vi "Periodic Tasks.vi"(8 "error in":errorcluster) -> ()   [LabVIEW 2017]
doc: "This VI runs in parallel to other robot code. It can contain as many user-defined periodic loops as you need. These can carry out PID or other sorts of timed response."
uses:
  <vilib>/Rock Robotics/WPI/Utilities/WPI_GetSetVariantRefNum.vi
  Robot Global Data.vi
  <vilib>/Rock Robotics/Network Tables/NT Write Number.vi
  <vilib>/Rock Robotics/Network Tables/NT Write Boolean.vi
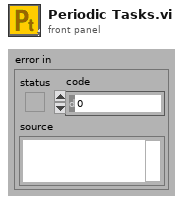
[diagram p1: front panel]
types:
  T1 = typedef "WPI_JoystickDevRef.ctl" = cluster{"Device":T2}
  T2 = typedef "WPI_JoystickDeviceEnum.ctl" = enum16{"USB 0", "USB 1", "USB 2", "USB 3", "USB 4", "USB 5"}
  T3 = typedef "WPI_GyroDevRef.ctl" = cluster{"DevStatus":errorcluster, "Analog Channel":T4, "Gain (VoltsPerDegree/Second)":dbl, "Gyro Type":enum16{"Analog", "XRS450"}, "Handle":i32, "SPI Bus":T5, "Device Found":bool, "Sample Rate":dbl, "Calibrate On Open":bool, "Offset":dbl}
  T4 = typedef "FPGA_AIChannel.ctl" = enum8{"AI 0", "AI 1", "AI 2", "AI 3", "AI MXP 0", "AI MXP 1", "AI MXP 2", "AI MXP 3", "Invalid"}
  T5 = typedef "spi_bus.ctl" = enum16{"SPI On-Board, CS0", "SPI On-Board, CS1", "SPI On-Board, CS2", "SPI On-Board, CS3", "SPI MXP", "Invalid"}
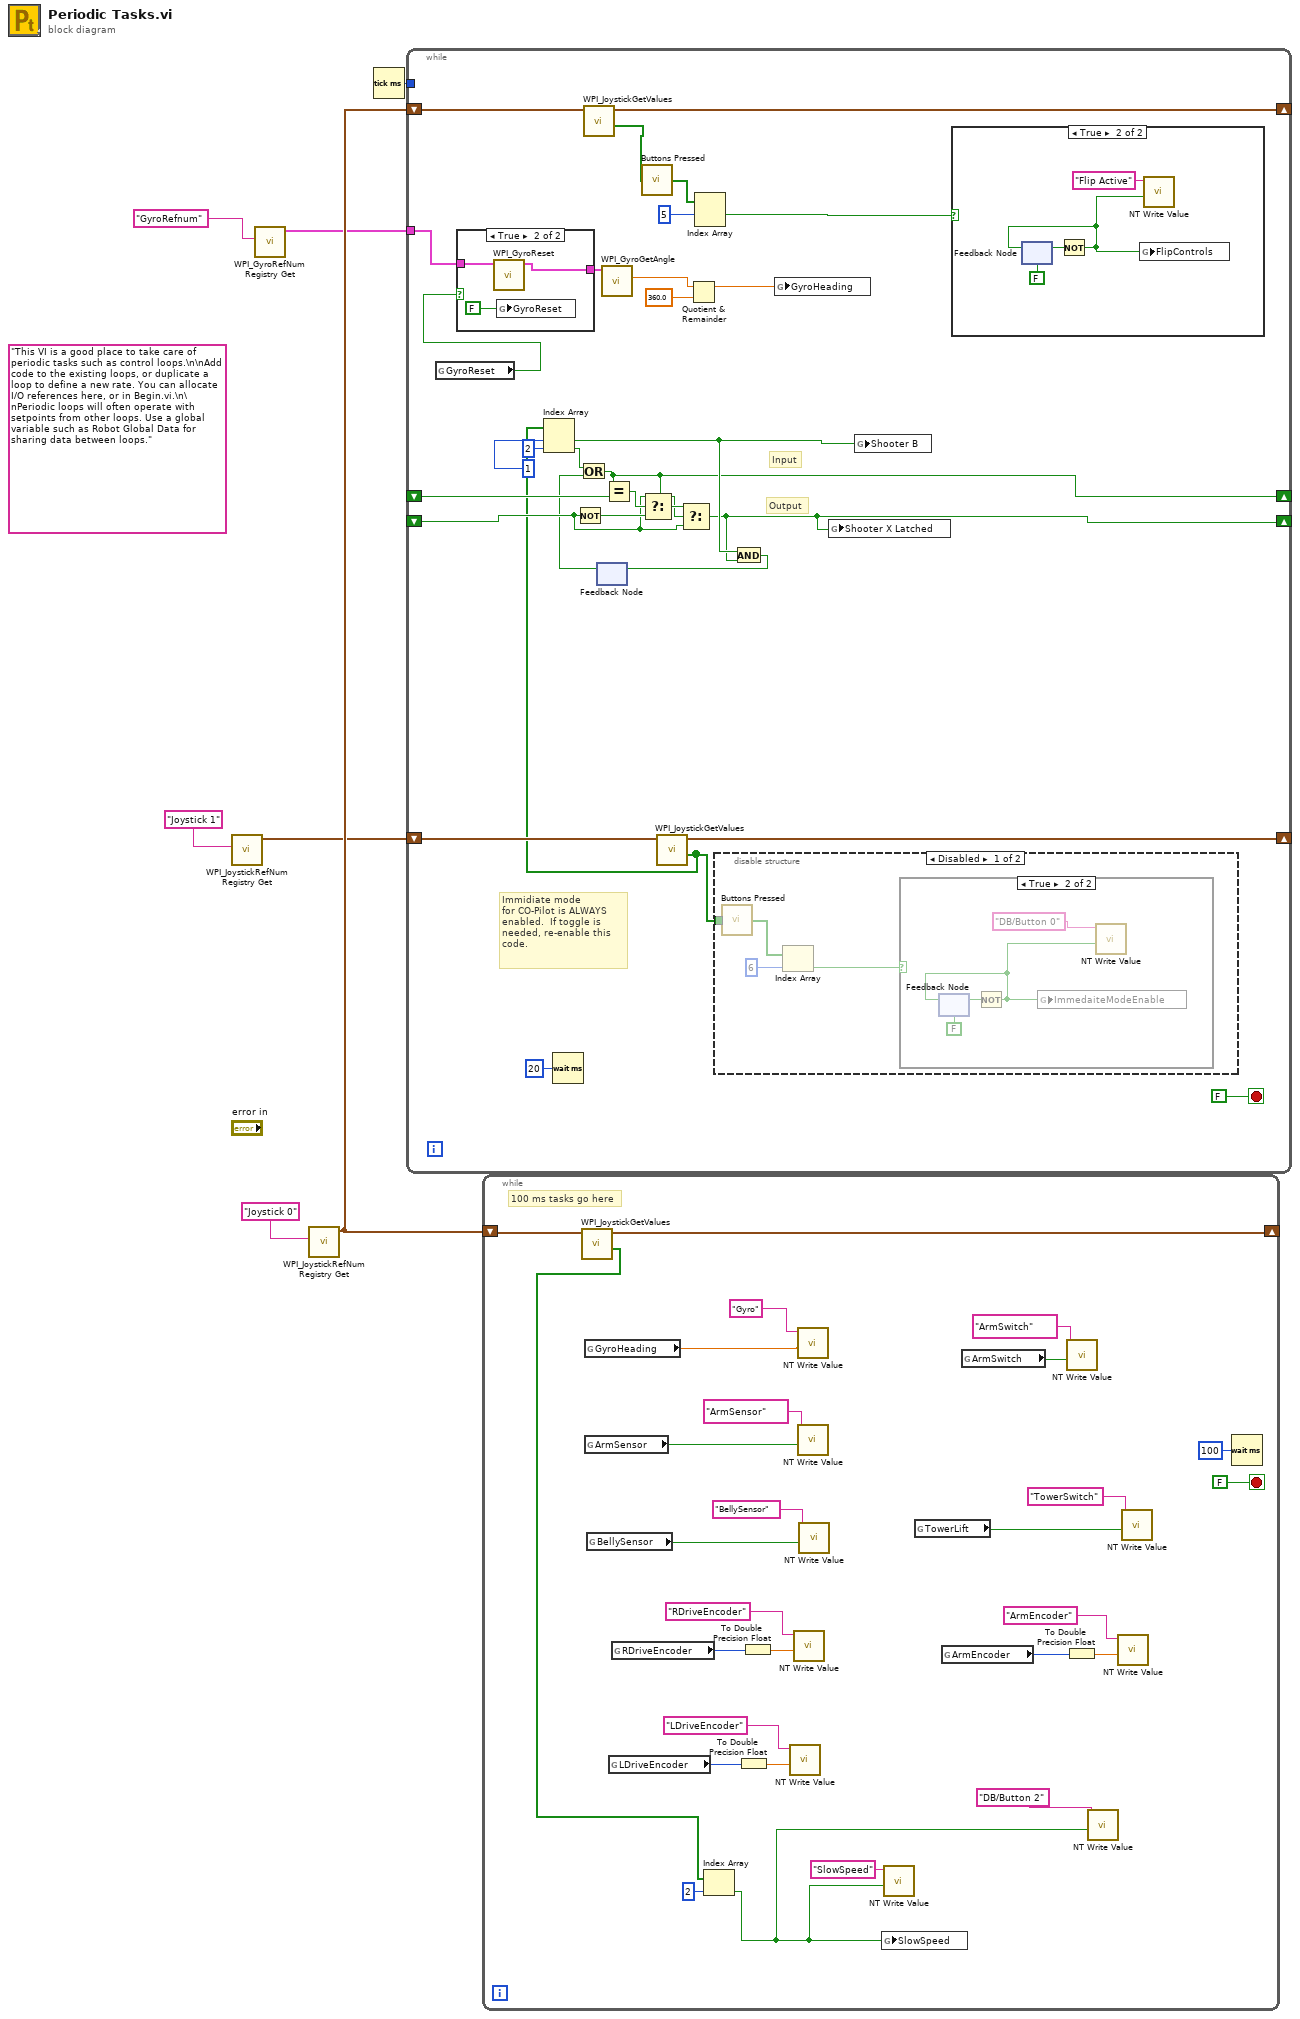
[diagram p0: block diagram]
diagram:
  (unwired) "This VI is a good place to take care of periodic tasks such as control loops.\n\nAdd code to the existing loops, or duplicate a loop to define a new rate. You can allocate I/O references here, or in Begin.vi.\n\nPeriodic loops will often operate with setpoints from other loops. Use a global variable such as Robot Global Data for sharing data between loops."
  n1 = call <vilib>:"WPI_JoystickRefNum Registry Get.vi"("refnum name"="Joystick 1") -> ("JoystickDevRef"=w1:T1)  [unwired: 1 in, 9 out]
  n2 = call <vilib>:"WPI_GyroRefNum Registry Get.vi"("refnum name"="GyroRefnum") -> ("GyroDevRef"=w3:T3)  [unwired: 9 in, 1 out]
  n3 = call <vilib>:"WPI_JoystickRefNum Registry Get.vi"("refnum name"="Joystick 0") -> ("JoystickDevRef"=w6:T1)  [unwired: 1 in, 9 out]
  n4 = Tick Count (ms)() -> (millisecond timer value=w5:u32)
  n5 = while {
    shift-right: [w32] -> _
    shift-left: w6 -> [w33]
    tunnel: w5 -> [_]
    tunnel: w3 -> [w25]
    shift-right: [w23] -> _
    shift-left: w1 -> [w24]
    shift-right: [w11] -> _
    shift-left: _ -> [w18]
    shift-right: [w12] -> _
    shift-left: _ -> [w17]
    stop <- FALSE stop-if-true
    # "Output"
    # "Input"
    # "Immidiate mode\nfor CO-Pilot is ALWAYS\nenabled.  If toggle is\nneeded, re-enable this\ncode."
    n6 = global read "Robot Global Data.vi" "GyroReset"() -> (w27:bool)
    n7 = case shown="True" w27 {
      tunnel: [w46 w48] -> w26
      tunnel: w25 -> [w46 w47]
      frame False {
      }
      frame True {
        n8 = call <vilib>:"WPI_GyroReset.vi"("GyroDevRef"=w47) -> ("GyroDevRef"=w48:T3)  [unwired: 9 in, 1 out]
        n9 = global write "Robot Global Data.vi" "GyroReset"(FALSE ("GyroReset")) -> ()
      }
    }
    n10 = Wait (ms)(milliseconds to wait=u32 20) -> ()  [unwired: 1 out]
    n11 = Not(x=w17) -> (.not. x?=w19:bool)
    n12 = call <vilib>:"WPI_JoystickGetValues.vi"("JoystickDevRef"=w33) -> ("Buttons"=w22:bool[], "JoystickDevRef"=w32:T1)  [unwired: 6 in, 3 out]
    n13 = feedback #1() -> (w8:bool)  [unwired: 1 in]
    n14 = call <vilib>:"WPI_GyroGetAngle.vi"("GyroDevRef"=w26) -> ("Angle"=w29:dbl)  [unwired: 6 in, 4 out]
    n15 = call "Buttons Pressed.vi"("Button Values"=w22) -> ("Button Presses"=w34:bool[])
    n16 = call <vilib>:"WPI_JoystickGetValues.vi"("JoystickDevRef"=w24) -> ("Buttons"=w16:bool[], "JoystickDevRef"=w23:T1)  [unwired: 6 in, 3 out]
    n17 = Index Array(array=w16, index #1=1 ("index"), index #2=2 ("index")) -> (element #1=w13:bool, element #2=w10:bool)
    n18 = Or(x=w10, y=w8) -> (x .or. y?=w11:bool)
    n19 = Equal?(x=w11, y=w18) -> (x = y?=w21:bool)
    n20 = Select(t=w17, s=w21, f=w19) -> (s? t:f=w20:bool)
    n21 = Select(t=w20, s=w11, f=w17) -> (s? t:f=w12:bool)
    n22 = Quotient & Remainder(x=w29, y=360.0) -> (x-y*floor(x/y)=w28:dbl)  [unwired: 1 out]
    n23 = Index Array(array=w34, index #1=5 ("index")) -> (element #1=w31:bool)  [unwired: 1 in, 1 out]
    n24 = disable-structure shown="Disabled" {
      disable-tunnel: w16 -> [w39 _]
      frame Disabled {
        n25 = call "Buttons Pressed.vi"("Button Values"=w39) -> ("Button Presses"=w41:bool[])
        n26 = Index Array(array=w41, index=6) -> (element=w38:bool)
        n27 = case shown="True" w38 {
          frame False {
          }
          frame True {
            n28 = feedback #2(FALSE) -> (w43:bool)
            n29 = Not(x=w43) -> (.not. x?=w42:bool)
            n30 = feedback-in #2(w42) -> ()
            n31 = global write "Robot Global Data.vi" "ImmedaiteModeEnable"(w42) -> ()
            n32 = call-poly <vilib>:"NT Write Value.vi"("Boolean"=w42, "Name"="DB/Button 0") -> ()  [unwired: 9 in, 1 out]
          }
        }
      }
      frame Enabled {
      }
    }
    n33 = And(x=w13, y=w12) -> (x .and. y?=w9:bool)
    n34 = feedback-in #1(w9) -> ()
    n35 = global write "Robot Global Data.vi" "GyroHeading"(w28) -> ()
    n36 = global write "Robot Global Data.vi" "Shooter X Latched"(w12) -> ()
    n37 = global write "Robot Global Data.vi" "Shooter B"(w13) -> ()
    n38 = case shown="True" w31 {
      frame False {
      }
      frame True {
        n39 = feedback #3(FALSE) -> (w51:bool)
        n40 = Not(x=w51) -> (.not. x?=w50:bool)
        n41 = feedback-in #3(w50) -> ()
        n42 = global write "Robot Global Data.vi" "FlipControls"(w50) -> ()
        n43 = call-poly <vilib>:"NT Write Value.vi"("Boolean"=w50, "Name"="Flip Active") -> ()  [unwired: 9 in, 1 out]
      }
    }
  }
  n44 = while {
    shift-right: [w78] -> _
    shift-left: w6 -> [w79]
    stop <- FALSE stop-if-true
    # "100 ms tasks go here"
    n45 = call <vilib>:"WPI_JoystickGetValues.vi"("JoystickDevRef"=w79) -> ("Buttons"=w58:bool[], "JoystickDevRef"=w78:T1)  [unwired: 6 in, 3 out]
    n46 = global read "Robot Global Data.vi" "GyroHeading"() -> (w77:dbl)
    n47 = global read "Robot Global Data.vi" "ArmSensor"() -> (w75:bool)
    n48 = global read "Robot Global Data.vi" "BellySensor"() -> (w72:bool)
    n49 = global read "Robot Global Data.vi" "LDriveEncoder"() -> (w62:i32)
    n50 = global read "Robot Global Data.vi" "RDriveEncoder"() -> (w70:i32)
    n51 = Index Array(array=w58, index=2) -> (element=w56:bool)
    n52 = To Double Precision Float(number=w62) -> (double precision float=w61:dbl)
    n53 = To Double Precision Float(number=w70) -> (double precision float=w69:dbl)
    n54 = call-poly <vilib>:"NT Write Value.vi"("Numeric"=w61, "Name"="LDriveEncoder") -> ()  [unwired: 9 in, 1 out]
    n55 = call-poly <vilib>:"NT Write Value.vi"("Numeric"=w69, "Name"="RDriveEncoder") -> ()  [unwired: 9 in, 1 out]
    n56 = call-poly <vilib>:"NT Write Value.vi"("Numeric"=w77, "Name"="Gyro") -> ()  [unwired: 9 in, 1 out]
    n57 = call-poly <vilib>:"NT Write Value.vi"("Boolean"=w75, "Name"="ArmSensor") -> ()  [unwired: 9 in, 1 out]
    n58 = call-poly <vilib>:"NT Write Value.vi"("Boolean"=w72, "Name"="BellySensor") -> ()  [unwired: 9 in, 1 out]
    n59 = global write "Robot Global Data.vi" "SlowSpeed"(w56) -> ()
    n60 = call-poly <vilib>:"NT Write Value.vi"("Boolean"=w56, "Name"="SlowSpeed") -> ()  [unwired: 9 in, 1 out]
    n61 = global read "Robot Global Data.vi" "TowerLift"() -> (w54:bool)
    n62 = global read "Robot Global Data.vi" "ArmEncoder"() -> (w67:i32)
    n63 = global read "Robot Global Data.vi" "ArmSwitch"() -> (w65:bool)
    n64 = call-poly <vilib>:"NT Write Value.vi"("Boolean"=w65, "Name"="ArmSwitch") -> ()  [unwired: 9 in, 1 out]
    n65 = To Double Precision Float(number=w67) -> (double precision float=w66:dbl)
    n66 = call-poly <vilib>:"NT Write Value.vi"("Boolean"=w56, "Name"="DB/Button 2") -> ()  [unwired: 9 in, 1 out]
    n67 = call-poly <vilib>:"NT Write Value.vi"("Numeric"=w66, "Name"="ArmEncoder") -> ()  [unwired: 9 in, 1 out]
    n68 = call-poly <vilib>:"NT Write Value.vi"("Boolean"=w54, "Name"="TowerSwitch") -> ()  [unwired: 9 in, 1 out]
    n69 = Wait (ms)(milliseconds to wait=u32 100) -> ()  [unwired: 1 out]
  }
